vi "DAQ_Initialization.vi"(7 "DO":tag="USB-6363/port0/line0:4", 8 "error in (no error)":errorcluster, 9 "Counter":tag="USB-6363/ctr0", 10 "Timing source":tag="OnboardClock", 11 "DO | Trigger":tag="/USB-6363/PFI12") -> (0 "error out":errorcluster)   [LabVIEW 2025]
uses:
  <vilib>/DAQmx/create/channels.llb/DAQmx Create Channel (CO-Pulse Generation-Time).vi
  <vilib>/DAQmx/create/channels.llb/DAQmx Create Channel (DO-Digital Output).vi
  <vilib>/DAQmx/configure/trigger.llb/DAQmx Start Trigger (Digital Edge).vi
  <vilib>/DAQmx/configure/timing.llb/DAQmx Timing (Sample Clock).vi
  <resource>/objmgr/daqmx.rc
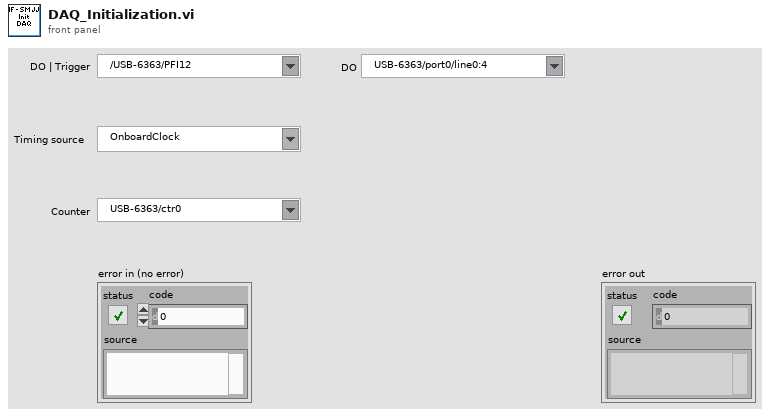
[diagram p1: front panel]
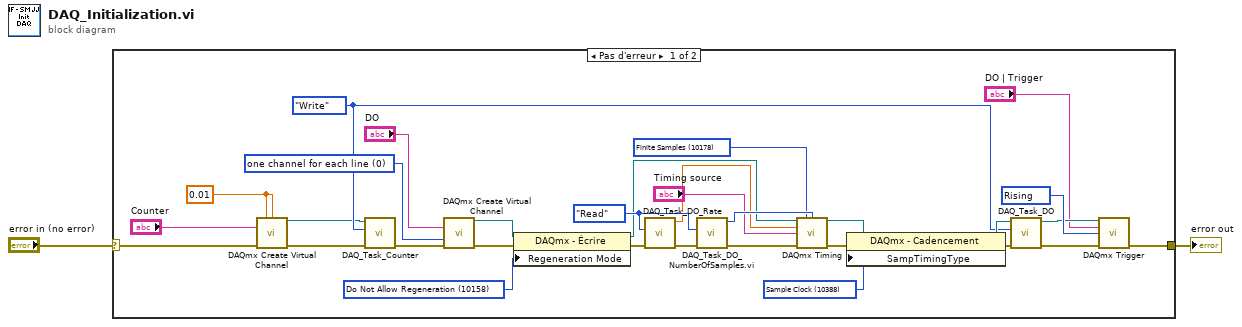
[diagram p0: block diagram]
diagram:
  n1 = case shown="Pas d'erreur" "error in (no error)" {
    selector: "error in (no error)" -> [w4 w34]
    tunnel: [w14 w34] -> w2
    frame No Error {
      w33 = 0 items=["one channel for each line", "one channel for all lines"] ("line grouping")
      w31 = enum16{"Write", "Read"}."Read" ("Action")
      w26 = 10388 items=["Sample Clock"=10388, "Burst Handshake"=12548, "Handshake"=10389, "Implicit"=10451, "On Demand"=10390, "Change Detection"=12504, "Pipelined Sample Clock"=14668] ("SampTimingType")
      w18 = 10178 items=["Finite Samples"=10178, "Continuous Samples"=10123] ("sample mode")
      w17 = 10158 items=["Allow Regeneration"=10097, "Do Not Allow Regeneration"=10158] ("RegenMode")
      w13 = 10280 items=["Rising"=10280, "Falling"=10171] ("edge")
      w12 = 0.01 ("low time")
      w15 = enum16{"Write", "Read"}."Write" ("Action")
      n2 = call-poly <vilib>:"DAQmx Create Virtual Channel.vi"("high time"=w12, "low time"=w12, "counter"="Counter", "error in"=w4) -> ("task out"=w8:refnum<k21>, "error out"=w7:errorcluster)  [unwired: 10 in]
      n3 = call "DAQ_Task_Counter.vi"("error in"=w7, "Action"=w15, "DAQ_Task_Counter"=w8) -> ("error out"=w9:errorcluster)  [unwired: 7 in, 1 out]
      n4 = call-poly <vilib>:"DAQmx Create Virtual Channel.vi"("lines"="DO", "line grouping"=w33, "error in"=w9) -> ("task out"=w21:refnum<k21>, "error out"=w20:errorcluster)  [unwired: 11 in]
      n5 = property class="DAQmx - Écrire"(reference=w21, error in=w20, "Regeneration Mode"=w17) -> (reference out=w16:refnum<k21>, error out=w27:errorcluster)
      n6 = call "DAQ_Task_DO_Rate.vi"("error in"=w27, "Action"=w31) -> ("error out"=w29:errorcluster, "DO_Rate"=w28:dbl)  [unwired: 8 in]
      n7 = call "DAQ_Task_DO_NumberOfSamples.vi.vi"("error in"=w29, "Action"=w31) -> ("error out"=w30:errorcluster, "Samples"=w32:i32)  [unwired: 8 in]
      n8 = call-poly <vilib>:"DAQmx Timing.vi"("task/channels in"=w16, "sample mode"=w18, "samples per channel"=w32, "rate"=w28, "source"="Timing source", "error in"=w30) -> ("task out"=w24:refnum<k21>, "error out"=w23:errorcluster)  [unwired: 8 in]
      n9 = property class="DAQmx - Cadencement"(reference=w24, error in=w23, "SampTimingType"=w26) -> (reference out=w25:refnum<k21>, error out=w22:errorcluster)
      n10 = call "DAQ_Task_DO.vi"("error in"=w22, "Action"=w15, "DAQ_Task_DO"=w25) -> ("error out"=w11:errorcluster, "DAQ_Task_DO"=w10:refnum<k21>)  [unwired: 7 in]
      n11 = call-poly <vilib>:"DAQmx Trigger.vi"("task/channels in"=w10, "source"="DO | Trigger", "edge"=w13, "error in"=w11) -> ("error out"=w14:errorcluster)  [unwired: 10 in, 1 out]
    }
    frame Error {
    }
  }
  "error out" <- w2
